vi "Configure Loss Compensation Table.vi"(4 "Frequency Array (0.0)":dbl[](array[numeric]), 5 "Port (1)":i32=1, 6 "Calibration Factor Array (0.0)":dbl[](array[numeric]), 7 "Channel (1)":i32=1, 8 "error in (no error)":errorcluster, 9 "Array Size (0)":i32, 11 "VISA resource name":refnum<visa-resource-name>) -> (0 "error out":errorcluster, 3 "VISA resource name out":refnum<visa-resource-name>)   [LabVIEW 2018, in "Agilent ENA Series.lvlib"]
doc: "Sets the loss compensation table for selected port of selected channel.\n\n<b>Note:</b>\nThis VI is not supported by the E5063A model."
uses:
  Agilent ENA Series.lvlib
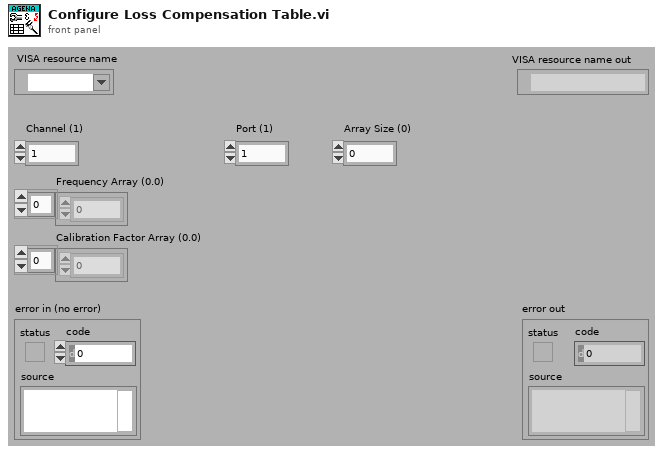
[diagram p1: front panel]
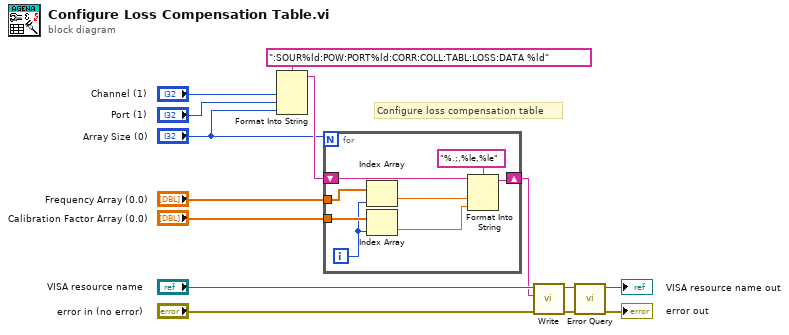
[diagram p0: block diagram]
diagram:
  # "Configure loss compensation table"
  n1 = Format Into String(format string=":SOUR%ld:POW:PORT%ld:CORR:COLL:TABL:LOSS:DATA %ld", "Channel (1)", "Port (1)", "Array Size (0)") -> (resulting string=w9:string)  [unwired: 2 in, 1 out]
  n2 = for {
    N: "Array Size (0)" -> [_]
    tunnel: "Frequency Array (0.0)" -> [w16]
    tunnel: "Calibration Factor Array (0.0)" -> [w19]
    shift-right: [w20] -> w8
    shift-left: w9 -> [w22]
    i -> [w15]
    n3 = Index Array(array=w16, index=w15) -> (element=w17:dbl)
    n4 = Index Array(array=w19, index=w15) -> (element=w18:dbl)
    n5 = Format Into String(format string="%.;,%le,%le", initial string=w22, w17, w18) -> (resulting string=w20:string)  [unwired: 1 in, 1 out]
  }
  n6 = call "Write.vi"("error in (no error)"="error in (no error)", "String ()"=w8, "VISA resource name"="VISA resource name") -> ("error out"=w3:errorcluster, "VISA resource name out"=w4:refnum<visa-resource-name>)  [unwired: 6 in, 1 out]
  n7 = call "Error Query.vi"("error in (no error)"=w3, "VISA resource name"=w4) -> ("error out"=→"error out":errorcluster, "VISA resource name out"=→"VISA resource name out":refnum<visa-resource-name>)  [unwired: 6 in, 2 out]
